vi "DM13 Hold.vi"(0 "Source Address":u8=27, 7 "Global?":bool) -> (4 "ID":u32 format="%.0x", 8 "Data":u8[](array[numeric]))   [LabVIEW 2019, in "J1939 Utilities.lvlib"]
uses:
  J1939 Utilities.lvlib
  Types/PGN Fields Cluster.ctl
  Convert J1939 ID to CAN Arb ID.vi
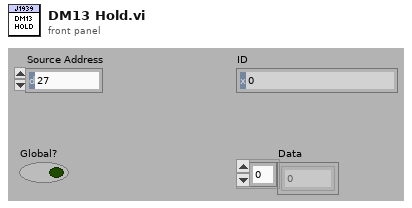
[diagram p1: front panel]
types:
  T1 = typedef "J1939 Utilities.lvlib/PGN Fields Cluster.ctl" = cluster{"Reserved Bit":u8, "Data page":u8, "PDU Format":u8, "PDU Specific":u8}
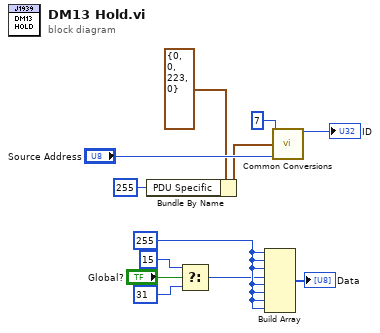
[diagram p0: block diagram]
diagram:
  w12 = u8 255
  n1 = Bundle By Name(cluster=T1 {"Reserved Bit"=0, "Data page"=0, "PDU Format"=223, "PDU Specific"=0} ("PGN Fields"), "PDU Specific"=u8 255) -> (w1:T1)
  n2 = Select(t=u8 15, s="Global?", f=u8 31) -> (s? t:f=w8:u8)
  n3 = Build Array(w12, w12, w12, w8, w12, w12, w12, w12) -> (→"Data":u8[])
  n4 = call-poly "Common Conversions.vi"("Priority"=u8 7, "PGN Fields"=w1, "Source Address"="Source Address") -> ("ID"=→"ID":u32)  [unwired: 11 in, 1 out]
